vi "isStringANumber.vi"(11 "Input String":string) -> (3 "Is A Number?":bool)   [LabVIEW 2016]
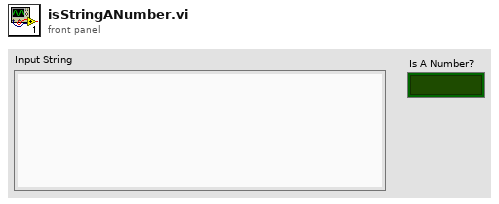
[diagram p1: front panel]
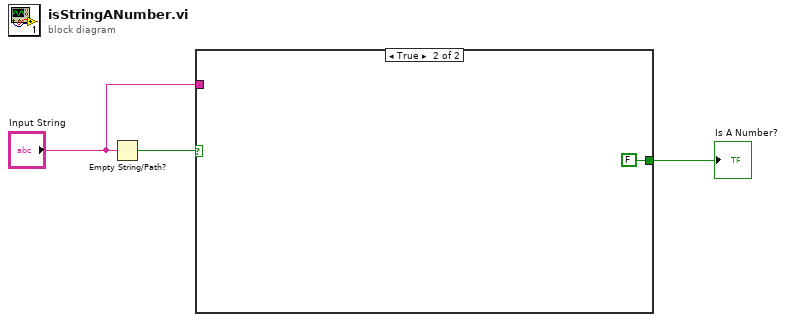
[diagram p0: block diagram]
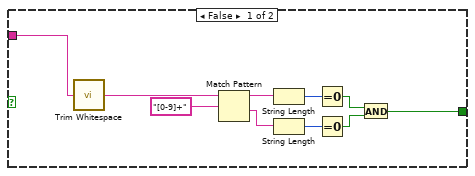
[diagram p2: hidden frame]
diagram:
  n1 = Empty String/Path?(string/path="Input String") -> (empty?=w2:bool)
  n2 = case shown="True" w2 {
    tunnel: [w5 FALSE] -> w3
    tunnel: "Input String" -> [w4 _]
    frame False {
      n3 = call <vilib>:"Trim Whitespace.vi"("string"=w4) -> ("trimmed string"=w6:string)  [unwired: 1 in]
      n4 = Match Pattern(string=w6, regular expression="[0-9]+") -> (before substring=w8:string, after substring=w9:string)  [unwired: 1 in, 2 out]
      n5 = String Length(string=w8) -> (length=w10:i32)
      n6 = String Length(string=w9) -> (length=w11:i32)
      n7 = Equal To 0?(x=w10) -> (x = 0?=w12:bool)
      n8 = Equal To 0?(x=w11) -> (x = 0?=w13:bool)
      n9 = And(x=w12, y=w13) -> (x .and. y?=w5:bool)
    }
    frame True {
    }
  }
  "Is A Number?" <- w3
